vi "Read (Statistical).vi"(0 "VISA resource name":refnum<visa-resource-name>, 1 "Sample Count (2)":i32=2, 2 "Output Mode (0: Fixed)":u16(ring) items=["Fixed", "Sweep", "List"], 5 "Statistical Operation (0: Mean)":u16(ring) items=["Mean", "Standard Deviation", "Maximum", "Minimum", "Peak to Peak"], 7 "Trace Data Source (0: Raw Data)":u16(ring) items=["Raw Data", "Math Data", "Limit Data"], 9 "Timeout (10000 ms)":i32=10000 format="%#.6g", 11 "error in (no error)":errorcluster) -> (4 "VISA resource name out":refnum<visa-resource-name>, 6 "Statistical Operation Results":dbl[](array[numeric]), 15 "error out":errorcluster)   [LabVIEW 2009, in "Keithley 24XX.lvlib"]
doc: "Initiates an acquisition and reads the result of the specified math operation."
uses:
  Keithley 24XX.lvlib
  Low Level/Fetch (Statistical).vi
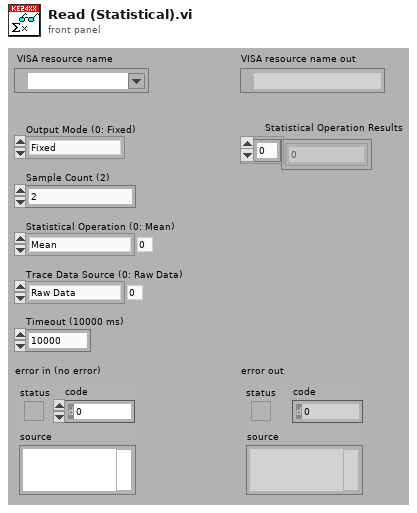
[diagram p1: front panel]
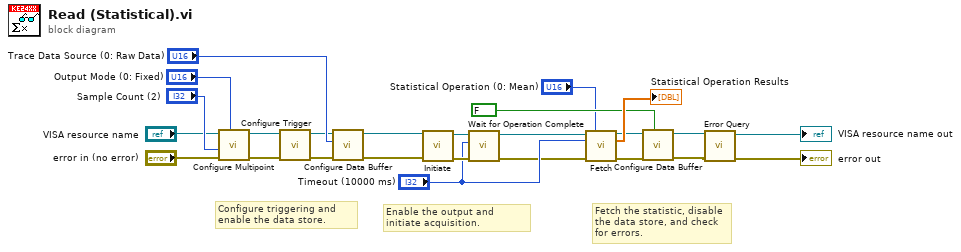
[diagram p0: block diagram]
diagram:
  # "Fetch the statistic, disable the data store, and check for errors."
  # "Enable the output and initiate acquisition."
  # "Configure triggering and enable the data store."
  n1 = call "Configure Multipoint.vi"("Output Mode (0: Fixed)"="Output Mode (0: Fixed)", "error in (no error)"="error in (no error)", "Trigger Count (1)"="Sample Count (2)", "VISA resource name"="VISA resource name") -> ("error out"=w18:errorcluster, "VISA resource name out"=w19:refnum<visa-resource-name>)  [unwired: 6 in]
  n2 = call "Configure Trigger.vi"("error in (no error)"=w18, "VISA resource name"=w19) -> ("error out"=w20:errorcluster, "VISA resource name out"=w21:refnum<visa-resource-name>)  [unwired: 8 in]
  n3 = call "Configure Data Buffer.vi"("error in (no error)"=w20, "Trace Data Source (0: Raw Data)"="Trace Data Source (0: Raw Data)", "VISA resource name"=w21) -> ("error out"=w2:errorcluster, "VISA resource name out"=w1:refnum<visa-resource-name>)  [unwired: 7 in]
  n4 = call "Initiate.vi"("error in (no error)"=w2, "VISA resource name"=w1) -> ("error out"=w12:errorcluster, "VISA resource name out"=w13:refnum<visa-resource-name>)  [unwired: 8 in]
  n5 = call "Wait for Operation Complete.vi"("error in (no error)"=w12, "Timeout (10000 ms)"="Timeout (10000 ms)", "VISA resource name"=w13) -> ("error out"=w3:errorcluster, "VISA resource name out"=w4:refnum<visa-resource-name>)  [unwired: 7 in]
  n6 = call-poly "Fetch.vi"("VISA resource name"=w4, "Statistical Operation (0: Mean)"="Statistical Operation (0: Mean)", "Timeout (10000 ms)"="Timeout (10000 ms)", "error in (no error)"=w3) -> ("VISA resource name out"=w10:refnum<visa-resource-name>, "Statistical Operation Results"=→"Statistical Operation Results":dbl[], "error out"=w11:errorcluster)  [unwired: 9 in]
  n7 = call "Configure Data Buffer.vi"("Enable Data Buffer (T: Enable)"=FALSE ("Enable Output (T: Enabled)"), "error in (no error)"=w11, "VISA resource name"=w10) -> ("error out"=w8:errorcluster, "VISA resource name out"=w9:refnum<visa-resource-name>)  [unwired: 7 in]
  n8 = call "Error Query.vi"("error in (no error)"=w8, "VISA resource name"=w9) -> ("error out"=→"error out":errorcluster, "VISA resource name out"=→"VISA resource name out":refnum<visa-resource-name>)  [unwired: 6 in, 2 out]
